vi "Open Variable Refs.vi"(1 "RT Data in":T1={"Device ref"=0, "Scan Period (uSec)"=10000, "Device Channels"={"Status"={"BD Refs"=[], "Length"=0, "FIFO Index"=0, "Data"=[]}, "Command"={"BD Refs"=[], "Data"=[], "Length"=0, "FIFO Index"=0}}, "Local Chassis"=[], "EtherCAT Masters"=[], "Async"={"Status"=refnum, "Command"=refnum, "Input FIFO"=refnum, "Input FIFO buffer"=[], "Output FIFO"=refnum, "Output FIFO buffer"=[], "Async VI Ref"=refnum}, "ECAT Reconfig"={"Reconfig Module Found"=FALSE, "VI Ref"=refnum, "Status"=refnum}, "Device Error"={"status"=FALSE, "code"=0, "source"=""}, "DeviceName"="", "PCLSync?"=FALSE} {"Device Channels"."Status"."BD Refs"."Data Reference" format="%.0x"; "Device Channels"."Command"."BD Refs"."Data Reference" format="%.0x"; "Local Chassis"."FPGA"."VS ref" format="%.0x"; "Local Chassis"."RSI Modules"."VS ref" format="%.0x"; "Local Chassis"."VS ref" format="%.0x"; "Device ref" format="%.0x"; "EtherCAT Masters"."DS402 Drive ECAT Slaves"."VS ref" format="%.0x"; "EtherCAT Masters"."REM IO ECAT Slaves"."VS ref" format="%.0x"; "EtherCAT Masters"."Generic EtherCAT Slaves"."VS ref" format="%.0x"; "EtherCAT Masters"."VS ref" format="%.0x"; "EtherCAT Masters"."EtherCAT Slaves"."FPGA"."VS ref" format="%.0x"; "EtherCAT Masters"."EtherCAT Slaves"."RSI Modules"."VS ref" format="%.0x"; "EtherCAT Masters"."EtherCAT Slaves"."VS ref" format="%.0x"}) -> (0 "RT Data out":T1={"Device ref"=0, "Scan Period (uSec)"=10000, "Device Channels"={"Status"={"BD Refs"=[], "Length"=0, "FIFO Index"=0, "Data"=[]}, "Command"={"BD Refs"=[], "Data"=[], "Length"=0, "FIFO Index"=0}}, "Local Chassis"=[], "EtherCAT Masters"=[], "Async"={"Status"=refnum, "Command"=refnum, "Input FIFO"=refnum, "Input FIFO buffer"=[], "Output FIFO"=refnum, "Output FIFO buffer"=[], "Async VI Ref"=refnum}, "ECAT Reconfig"={"Reconfig Module Found"=FALSE, "VI Ref"=refnum, "Status"=refnum}, "Device Error"={"status"=FALSE, "code"=0, "source"=""}, "DeviceName"="", "PCLSync?"=FALSE} {"Device Channels"."Status"."BD Refs"."Data Reference" format="%.0x"; "Device Channels"."Command"."BD Refs"."Data Reference" format="%.0x"; "Local Chassis"."FPGA"."VS ref" format="%.0x"; "Local Chassis"."RSI Modules"."VS ref" format="%.0x"; "Local Chassis"."VS ref" format="%.0x"; "Device ref" format="%.0x"; "EtherCAT Masters"."DS402 Drive ECAT Slaves"."VS ref" format="%.0x"; "EtherCAT Masters"."REM IO ECAT Slaves"."VS ref" format="%.0x"; "EtherCAT Masters"."Generic EtherCAT Slaves"."VS ref" format="%.0x"; "EtherCAT Masters"."VS ref" format="%.0x"; "EtherCAT Masters"."EtherCAT Slaves"."FPGA"."VS ref" format="%.0x"; "EtherCAT Masters"."EtherCAT Slaves"."RSI Modules"."VS ref" format="%.0x"; "EtherCAT Masters"."EtherCAT Slaves"."VS ref" format="%.0x"})   [LabVIEW 2016, in "Scan Engine Custom Device.lvlib"]
uses:
  Scan Engine Custom Device.lvlib
  Type Defs/RT Data.ctl
  <vilib>/NI Veristand/Custom Device API/Custom Device Item Ref.ctl
  Type Defs/Device Channels.ctl
  Type Defs/Output Data.ctl
  <vilib>/NI Veristand/Custom Device API/Block Data Reference.ctl
  <vilib>/NI Veristand/Custom Device API/Data Reference.ctl
  Type Defs/Input Data.ctl
  Type Defs/Local Chassis Data.ctl
  Type Defs/RSI Module Data.ctl
  Type Defs/Open Module IOVs.ctl
  Modules.lvlibp/RSI Module/RSI Module.lvclass
  Modules.lvlibp/RSI Module/Module Models.ctl
  Modules.lvlibp/RSI Module/Channel Type.ctl
  Type Defs/Module Config Data.ctl
  Type Defs/Mixed IO.ctl
  Type Defs/FPGA Data.ctl
  Type Defs/UDV Data.ctl
  Type Defs/UDV Data Type.ctl
  Type Defs/FXP Config.ctl
  Type Defs/Mod Size Indexes.ctl
  Type Defs/EtherCAT Master Data.ctl
  Type Defs/EtherCAT Slave Data.ctl
  Type Defs/Generic ECAT Slave RT-Data-Array.ctl
  Type Defs/Generic ECAT Slave Data Cluster.ctl
  Type Defs/Generic ECAT Slave IOV Cluster.ctl
  Type Defs/REM IO ECAT Slave RT-Data-Array.ctl
  Type Defs/REM IO ECAT Slave Data Cluster.ctl
  Type Defs/REM IO ECAT Slave IOV Cluster.ctl
  Type Defs/DS402 Drive ECAT Slave RT-Data-Array.ctl
  Type Defs/DS402 Drive ECAT Slave Data Cluster.ctl
  Type Defs/DS402 Drive ECAT Slave IOV Cluster.ctl
  Type Defs/DS402 Drive ECAT Slave Action IOV Cluster.ctl
  Type Defs/Async Data.ctl
  Type Defs/Async Status.ctl
  Type Defs/Async State.ctl
  Type Defs/Async Command.ctl
  Type Defs/ECAT Reconfig Data.ctl
  Type Defs/ECAT Reconfig Status.ctl
  Type Defs/ECAT Reconfig State.ctl
  <vilib>/NI Veristand/Custom Device API/Custom Device API.lvlib
types:
  T1 = typedef "Scan Engine Custom Device.lvlib/RT Data.ctl" = cluster{"Device ref":T2, "Scan Period (uSec)":u32, "Device Channels":T3, "Local Chassis":T8[], "EtherCAT Masters":T20[], "Async":T32, "ECAT Reconfig":T33, "Device Error":errorcluster, "DeviceName":string, "PCLSync?":bool}
  T2 = typedef "Custom Device API.lvlib/Custom Device Item Ref.ctl" = u64
  T3 = typedef "Scan Engine Custom Device.lvlib/Device Channels.ctl" = cluster{"Status":T4, "Command":T7}
  T4 = typedef "Scan Engine Custom Device.lvlib/Output Data.ctl" = cluster{"BD Refs":T5[], "Length":i32, "FIFO Index":i32, "Data":dbl[]}
  T5 = typedef "Custom Device API.lvlib/Block Data Reference.ctl" = cluster{"Data Reference":T6, "Offset":u64, "Length":u64}
  T6 = typedef "Custom Device API.lvlib/Data Reference.ctl" = i32
  T7 = typedef "Scan Engine Custom Device.lvlib/Input Data.ctl" = cluster{"BD Refs":T5[], "Data":dbl[], "Length":i32, "FIFO Index":i32}
  T8 = typedef "Scan Engine Custom Device.lvlib/Local Chassis Data.ctl" = cluster{"VS ref":T2, "RSI Modules":T9[], "FPGA":T15[], "Input Mod Size Idxs":T19, "Output Modules":i32[], "MixedIO Mod Size Idxs":T19}
  T9 = typedef "Scan Engine Custom Device.lvlib/RSI Module Data.ctl" = cluster{"VS ref":T2, "IOV ref":refnum<k21>, "Open Mod refs":T10, "Module DVR":refnum<data-value>, "Slot":u32, "Model":T11, "Channel Type":T12, "EtherCAT?":bool, "CDInput Data":T7, "CDOutput Data":T4, "Module Config Data":T13, "Mixed IO":T14}
  T10 = typedef "Scan Engine Custom Device.lvlib/Open Module IOVs.ctl" = cluster{"Analog Read":refnum<k21>, "Digital Read":refnum<k21>, "Analog Write":refnum<k21>, "Digital Write":refnum<k21>}
  T11 = typedef "Modules.lvlibp/RSI Module.lvclass/Module Models.ctl" = enum16{"Empty", "NI 9201", "NI 9203", "NI 9205", "NI 9206", "NI 9207", "NI 9208", "NI 9211", "NI 9212", "NI 9213", "NI 9214", "NI 9215", "NI 9217", "NI 9219", "NI 9220", "NI 9221", "NI 9222", "NI 9223", "NI 9225", "NI 9227", "NI 9229", "NI 9233", "NI 9234", "NI 9235", "NI 9236", "NI 9237", "NI 9239", "NI 9242", "NI 9244", "NI 9263", "NI 9264", "NI 9265", "NI 9269", "NI 9375", "NI 9401", "NI 9402", "NI 9403", "NI 9411", "NI 9421", "NI 9422", "NI 9423", "NI 9425", "NI 9426", "NI 9435", "NI 9437", "NI 9472", "NI 9474", "NI 9475", "NI 9476", "NI 9477", "NI 9478", "NI 9481", "NI 9482", "NI 9485"}
  T12 = typedef "Modules.lvlibp/RSI Module.lvclass/Channel Type.ctl" = enum16{"Analog", "Digital"}
  T13 = typedef "Scan Engine Custom Device.lvlib/Module Config Data.ctl" = cluster{"Configurable?":bool, "Config Block Data Refs":T5[], "Config Data DVR":refnum<data-value>, "Previous Values":dbl[], "Local Reconfig VI Ref":refnum<vi>}
  T14 = typedef "Scan Engine Custom Device.lvlib/Mixed IO.ctl" = cluster{"Input Channel Indices":i32[], "Input Buffer":dbl[]}
  T15 = typedef "Scan Engine Custom Device.lvlib/FPGA Data.ctl" = cluster{"VS ref":T2, "IOV ref":refnum<k21>, "FPGA Target":enum16{"Local", "EtherCAT"}, "Product Code":u32, "Bitfile Signature":string, "Bitfile Path (RT)":path, "FPGA Session":u32, "Input Data":T7, "Output Data":T4, "UDVs":cluster{"From FPGA":T16[], "To FPGA":T16[]}}
  T16 = typedef "Scan Engine Custom Device.lvlib/UDV Data.ctl" = cluster{"VS ref":T2, "IOV Ref":refnum<k21>, "Name":string, "UDV Data Type":T17, "Supported Type?":bool, "FXP Config":T18, "FXP VI Ref":refnum<vi>}
  T17 = typedef "Scan Engine Custom Device.lvlib/UDV Data Type.ctl" = enum16{"Boolean", "Fixed Point", "Int8", "Int16", "Int32", "Int64", "U32 Bit Field", "UInt8", "UInt16", "UInt32", "UInt64", "Other"}
  T18 = typedef "Scan Engine Custom Device.lvlib/FXP Config.ctl" = cluster{"signed":bool, "size":u32, "integersize":i32}
  T19 = typedef "Scan Engine Custom Device.lvlib/Mod Size Indexes.ctl" = cluster{"4":i32[], "8":i32[], "16":i32[], "32":i32[], "other":i32[]}
  T20 = typedef "Scan Engine Custom Device.lvlib/EtherCAT Master Data.ctl" = cluster{"VS ref":T2, "IOV ref":refnum<k21>, "Master ID":u32, "Cyclic Data Bandwidth":u32, "EtherCAT Slaves":T21[], "Generic EtherCAT Slaves":T22, "REM IO ECAT Slaves":T25, "DS402 Drive ECAT Slaves":T28}
  T21 = typedef "Scan Engine Custom Device.lvlib/EtherCAT Slave Data.ctl" = cluster{"VS ref":T2, "IOV ref":refnum<k21>, "Position Address":u16, "RSI Modules":T9[], "FPGA":T15[], "Input Mod Size Idxs":T19, "Output Modules":i32[], "MixedIO Mod Size Idxs":T19}
  T22 = typedef "Scan Engine Custom Device.lvlib/Generic ECAT Slave RT-Data-Array.ctl" = T23[]
  T23 = typedef "Scan Engine Custom Device.lvlib/Generic ECAT Slave Data Cluster.ctl" = cluster{"VS ref":T2, "IOV ref":refnum<k21>, "Position Address":u16, "I/O Imput Vars ":T24[], "I/O Output Vars":T24[], "I/O Input Data":T7, "I/O Output Data":T4}
  T24 = typedef "Scan Engine Custom Device.lvlib/Generic ECAT Slave IOV Cluster.ctl" = cluster{"VS ref":T2, "IOV Ref":refnum<k21>, "Name":string, "UDV Data Type":T17}
  T25 = typedef "Scan Engine Custom Device.lvlib/REM IO ECAT Slave RT-Data-Array.ctl" = T26[]
  T26 = typedef "Scan Engine Custom Device.lvlib/REM IO ECAT Slave Data Cluster.ctl" = cluster{"VS ref":T2, "IOV ref":refnum<k21>, "Position Address":u16, "I/O Imput Vars ":T27[], "I/O Output Vars":T27[], "I/O Input Data":T7, "I/O Output Data":T4}
  T27 = typedef "Scan Engine Custom Device.lvlib/REM IO ECAT Slave IOV Cluster.ctl" = cluster{"VS ref":T2, "IOV Ref":refnum<k21>, "Name":string, "UDV Data Type":T17, "Scaling Factor":dbl}
  T28 = typedef "DS402 Drive ECAT Slave RT-Data-Array.ctl" = T29[]
  T29 = typedef "Scan Engine Custom Device.lvlib/DS402 Drive ECAT Slave Data Cluster.ctl" = cluster{"VS ref":T2, "IOV ref":refnum<k21>, "Position Address":u16, "I/O Input Vars ":T30[], "I/O Output Vars":T30[], "I/O Input Data":T7, "I/O Output Data":T4, "DS402 IOV":T31}
  T30 = typedef "Scan Engine Custom Device.lvlib/DS402 Drive ECAT Slave IOV Cluster.ctl" = cluster{"VS ref":T2, "IOV Ref":refnum<k21>, "Name":string, "UDV Data Type":T17, "Scaling Factor":dbl, "IOV":bool, "VS data Index":i32}
  T31 = typedef "Scan Engine Custom Device.lvlib/DS402 Drive ECAT Slave Action IOV Cluster.ctl" = cluster{"Control Word":refnum<k21>, "Status Word":refnum<k21>}
  T32 = typedef "Scan Engine Custom Device.lvlib/Async Data.ctl" = cluster{"Status":refnum<queue>, "Command":refnum<queue>, "Input FIFO":refnum<k33>, "Input FIFO buffer":dbl[], "Output FIFO":refnum<k33>, "Output FIFO buffer":dbl[], "Async VI Ref":refnum<vi>}
  T33 = typedef "Scan Engine Custom Device.lvlib/ECAT Reconfig Data.ctl" = cluster{"Reconfig Module Found":bool, "VI Ref":refnum<vi>, "Status":refnum<queue>}
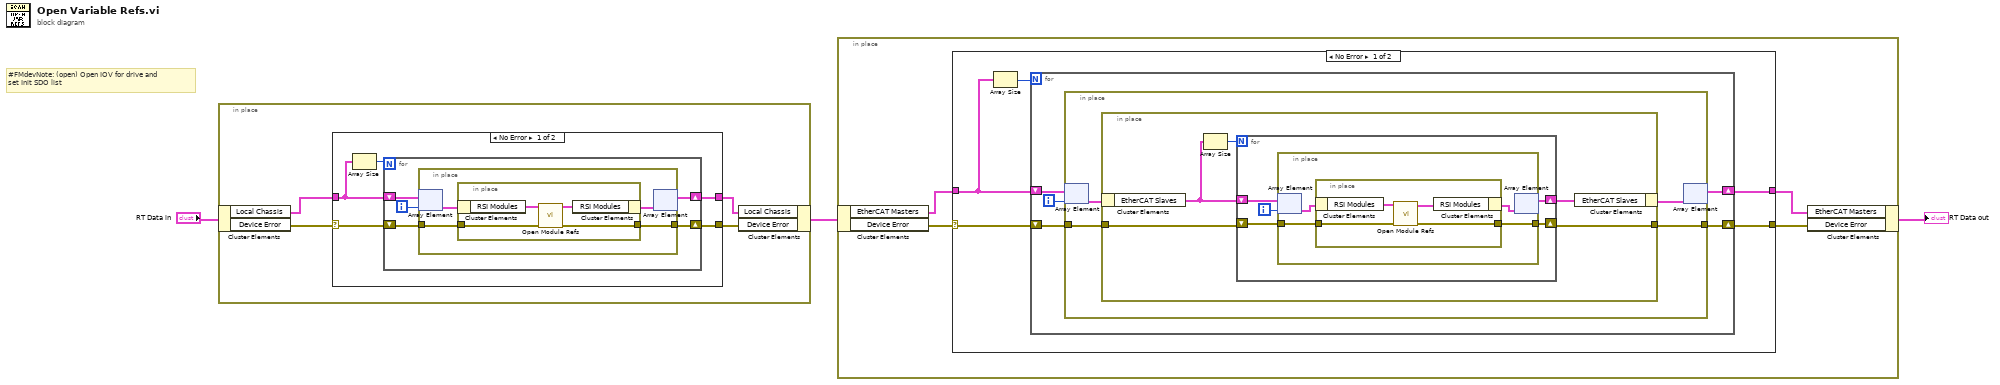
[diagram p0: block diagram]
diagram:
  # "#FMdevNote: (open) Open IOV for drive and \nset Init SDO list"
  n1 = in-place {
    n2 = in-place-cluster #1("RT Data in") -> ("Local Chassis"=w6:T8[], "Device Error"=w7:errorcluster)
    n3 = case shown="No Error" w7 {
      selector: w7 -> [w10 w27]
      tunnel: [w8 w27] -> w5
      tunnel: w6 -> [w11 w26]
      tunnel: [w9 w26] -> w4
      frame No Error {
        n4 = Array Size(array=w11) -> (size(s)=w12:i32)
        n5 = for {
          N: w12 -> [_]
          shift-right: [w13] -> w9
          shift-left: w11 -> [w17]
          shift-right: [w14] -> w8
          shift-left: w10 -> [w15]
          i -> [w16]
          n6 = in-place {
            in-place-border: w15 -> [w19]
            in-place-border: [w18] -> w14
            n7 = in-place-array #2(w17, w16) -> (w21:T8)
            n8 = in-place {
              in-place-border: w19 -> [w25]
              in-place-border: [w24] -> w18
              n9 = in-place-cluster #3(w21) -> ("RSI Modules"=w23:T9[])
              n10 = call "Open Module Refs.vi"("error in (no error)"=w25, "RSI Modules in"=w23) -> ("error out"=w24:errorcluster, "RSI Modules out"=w22:T9[])  [unwired: 8 in]
              n11 = in-place-cluster #3("RSI Modules"=w22) -> (w20:T8)
            }
            n12 = in-place-array #2(w20) -> (w13:T8[])  [unwired: 1 out]
          }
        }
      }
      frame Error {
      }
    }
    n13 = in-place-cluster #1("Local Chassis"=w4, "Device Error"=w5) -> (w2:T1)
  }
  n14 = in-place {
    n15 = in-place-cluster #4(w2) -> ("EtherCAT Masters"=w30:T20[], "Device Error"=w31:errorcluster)
    n16 = case shown="No Error" w31 {
      selector: w31 -> [w32 w65]
      tunnel: [w33 w65] -> w29
      tunnel: w30 -> [w35 w64]
      tunnel: [w34 w64] -> w28
      frame No Error {
        n17 = Array Size(array=w35) -> (size(s)=w36:i32)
        n18 = for {
          N: w36 -> [_]
          shift-right: [w38] -> w33
          shift-left: w32 -> [w39]
          shift-right: [w37] -> w34
          shift-left: w35 -> [w41]
          i -> [w40]
          n19 = in-place {
            in-place-border: w39 -> [w44]
            in-place-border: [w43] -> w38
            n20 = in-place-array #5(w41, w40) -> (w45:T20)
            n21 = in-place {
              in-place-border: w44 -> [w46]
              in-place-border: [w48] -> w43
              n22 = in-place-cluster #6(w45) -> ("EtherCAT Slaves"=w50:T21[])
              n23 = Array Size(array=w50) -> (size(s)=w49:i32)
              n24 = for {
                N: w49 -> [_]
                shift-right: [w52] -> w48
                shift-left: w46 -> [w53]
                shift-right: [w51] -> w47
                shift-left: w50 -> [w55]
                i -> [w54]
                n25 = in-place {
                  in-place-border: w53 -> [w58]
                  in-place-border: [w57] -> w52
                  n26 = in-place-array #7(w55, w54) -> (w59:T21)
                  n27 = in-place {
                    in-place-border: w58 -> [w63]
                    in-place-border: [w62] -> w57
                    n28 = in-place-cluster #8(w59) -> ("RSI Modules"=w61:T9[])
                    n29 = call "Open Module Refs.vi"("error in (no error)"=w63, "RSI Modules in"=w61) -> ("error out"=w62:errorcluster, "RSI Modules out"=w60:T9[])  [unwired: 8 in]
                    n30 = in-place-cluster #8("RSI Modules"=w60) -> (w56:T21)
                  }
                  n31 = in-place-array #7(w56) -> (w51:T21[])  [unwired: 1 out]
                }
              }
              n32 = in-place-cluster #6("EtherCAT Slaves"=w47) -> (w42:T20)
            }
            n33 = in-place-array #5(w42) -> (w37:T20[])  [unwired: 1 out]
          }
        }
      }
      frame Error {
      }
    }
    n34 = in-place-cluster #4("EtherCAT Masters"=w28, "Device Error"=w29) -> (→"RT Data out":T1)
  }
